vi "OAT Compensate Even Angle Signal (Even Angle Ref, 1 Channel).vi"(0 "even-angle signal":cluster{"r0":dbl, "dr":dbl, "Y":dbl[]}={"r0"=0.0, "dr"=1.0, "Y"=[]} {"r0" format="%.2p"; "dr" format="%.2p"; "Y" format="%.2f"}, 2 "reset? (F)":bool, 5 "even-angle reference":cluster{"r0":dbl, "dr":dbl, "Y":dbl[]}={"r0"=0.0, "dr"=1.0, "Y"=[]} {"r0" format="%.2p"; "dr" format="%.2p"; "Y" format="%.2f"}, 7 "even-angle position info":T1, 9 "speed profile":T2 {"speed [RPM]" format="%.2f"; "time [s]" format="%.2f"}, 11 "error in (no error)":errorcluster) -> (4 "compensated even-angle signal":cluster{"r0":dbl, "dr":dbl, "Y":dbl[]}={"r0"=0.0, "dr"=1.0, "Y"=[]} {"r0" format="%.2p"; "dr" format="%.2p"; "Y" format="%.2f"}, 6 "actual even-angle reference":cluster{"r0":dbl, "dr":dbl, "Y":dbl[]}={"r0"=0.0, "dr"=1.0, "Y"=[]} {"r0" format="%.2p"; "dr" format="%.2p"; "Y" format="%.2f"}, 8 "even-angle position info out":T1, 15 "error out":errorcluster)   [LabVIEW 2017, in "SoundVib_RefDataProcess.lvlib"]
doc: "Compensates an even-angle signal. You can use the <B>compensated even-angle signal</B> output to display unfiltered orbit and timebase plots with the runout pattern removed. Wire data to the <B>even-angle signal</B> input to determine the polymorphic instance to use or manually select the instance."
uses:
  <vilib>/addons/Sound and Vibration/Order Analysis/Referece Data Processing/SoundVib_RefDataProcess.lvlib
  <vilib>/addons/Sound and Vibration/Order Analysis/Misc/OAT Position Info.ctl
  <vilib>/addons/Sound and Vibration/Order Analysis/Tach Process/SubVIs/speed profile.ctl
  <vilib>/addons/Sound and Vibration/Order Analysis/Resample Order Tracking/SoundVib_Resampling.lvlib
  <vilib>/addons/Sound and Vibration/Order Analysis/Tach Process/SoundVib_TachProcess.lvlib
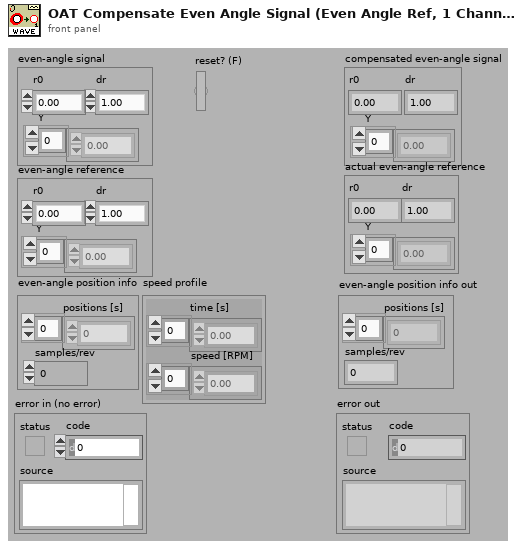
[diagram p1: front panel]
types:
  T1 = typedef "OAT Position Info.ctl" = cluster{"positions [s]":dbl[], "samples/rev":dbl}
  T2 = typedef "SoundVib_TachProcess.lvlib/speed profile.ctl" = cluster{"time [s]":dbl[], "speed [RPM]":dbl[]}
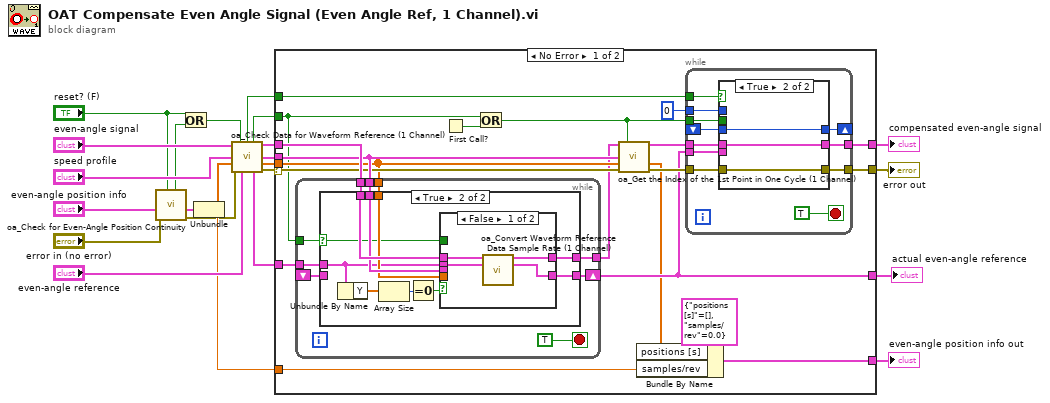
[diagram p0: block diagram]
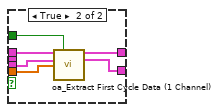
[diagram p3: hidden frame]
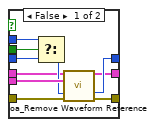
[diagram p4: hidden frame]
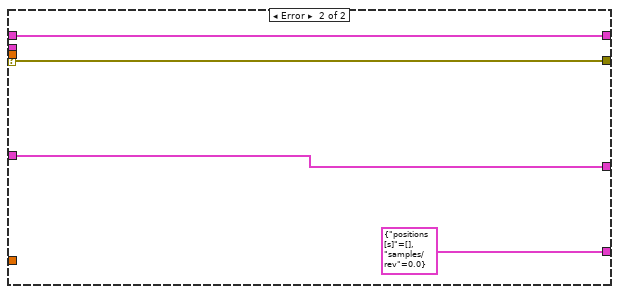
[diagram p5: hidden frame]
diagram:
  n1 = call <vilib>:"oa_Check for Even-Angle Position Continuity.vi"("reset in"="reset? (F)", "error in (no error)"="error in (no error)", "even-angle position info"="even-angle position info") -> ("error out"=w6:errorcluster, "even-angle position info dup"=w5:T1, "position not continuous"=w2:bool)  [unwired: 6 in]
  n2 = Or(x="reset? (F)", y=w2) -> (x .or. y?=w1:bool)
  n3 = Unbundle(w5) -> ("positions [s]"=w14:dbl[], "samples/rev"=w9:dbl)
  n4 = call <vilib>:"oa_Check Data for Waveform Reference (1 Channel).vi"("resampled signal"="even-angle signal", "reset? (True)"=w1, "speed profile"="speed profile", "interpolated pulse positions"=w14, "error in (no error)"=w6, "even angle reference in"="even-angle reference") -> ("empty signal?"=w10:bool, "reset"=w13:bool, "resampled signal out"=w20:cluster{"r0":dbl, "dr":dbl, "Y":dbl[]}, "speed profile out"=w19:T2, "interpolated pulse positions out"=w18:dbl[], "even angle reference out"=w11:cluster{"r0":dbl, "dr":dbl, "Y":dbl[]}, "error out"=w21:errorcluster)  [unwired: 2 in, 1 out]
  n5 = case shown="No Error" w21 {
    selector: w21 -> [w41 w102]
    tunnel: w20 -> [w43 w101]
    tunnel: w19 -> [w42 _]
    tunnel: w18 -> [w35 _]
    tunnel: [w37 w101] -> w17
    tunnel: [w34 w100] -> w16
    tunnel: [w38 w102] -> w15
    tunnel: w13 -> [w32 _]
    tunnel: w11 -> [w30 w100]
    tunnel: w10 -> [w29 _]
    tunnel: w9 -> [w27 _]
    tunnel: [w25 T1 {"positions [s]"=[], "samples/rev"=0.0} ("even angle position info")] -> w8
    frame No Error {
      n6 = while {
        tunnel: w43 -> [w52]
        tunnel: w42 -> [w51]
        tunnel: w32 -> [w46]
        tunnel: [w50] -> w24
        tunnel: w35 -> [w49]
        shift-right: [w47] -> w34
        shift-left: _ -> [w45]
        tunnel: w30 -> [w44]
        stop <- TRUE stop-if-true
        n7 = case shown="True" w46 {
          selector: w46 -> [_ w56]
          tunnel: w52 -> [w53 w64]
          tunnel: w51 -> [_ w63]
          tunnel: [w53 w59] -> w50
          tunnel: w49 -> [_ w58]
          tunnel: [w54 w57] -> w47
          tunnel: w45 -> [w54 _]
          tunnel: w44 -> [_ w55]
          frame False {
          }
          frame True {
            n8 = Unbundle By Name(w55) -> ("Y"=w62:dbl[])
            n9 = Array Size(array=w62) -> (size(s)=w61:i32)
            n10 = Equal To 0?(x=w61) -> (x = 0?=w60:bool)
            n11 = case shown="False" w60 {
              tunnel: w55 -> [w67 _]
              tunnel: [w66 w69] -> w57
              tunnel: w64 -> [w68 w74]
              tunnel: w56 -> [_ w73]
              tunnel: w63 -> [_ w72]
              tunnel: [w65 w70] -> w59
              tunnel: w58 -> [_ w71]
              frame False {
                n12 = call <vilib>:"oa_Convert Waveform Reference Data Sample Rate (1 Channel).vi"("resampled signal"=w68, "baseline in"=w67) -> ("resampled signal dup"=w65:cluster{"r0":dbl, "dr":dbl, "Y":dbl[]}, "baseline in out"=w66:cluster{"r0":dbl, "dr":dbl, "Y":dbl[]})  [unwired: 11 in, 1 out]
              }
              frame True {
                n13 = call <vilib>:"oa_Extract First Cycle Data (1 Channel).vi"("resampled signal"=w74, "reset? (True)"=w73, "speed profile"=w72, "interpolated pulse positions"=w71) -> ("resampled signal out"=w70:cluster{"r0":dbl, "dr":dbl, "Y":dbl[]}, "waveform reference data"=w69:cluster{"r0":dbl, "dr":dbl, "Y":dbl[]})  [unwired: 9 in, 1 out]
              }
            }
          }
        }
      }
      n14 = First Call?() -> (First Call?: T/F=w31:bool)
      n15 = Or(x=w32, y=w31) -> (x .or. y?=w33:bool)
      n16 = call <vilib>:"oa_Get the Index of the 1st Point in One Cycle (1 Channel).vi"("resampled signal"=w24, "reset? (True)"=w33, "speed profile"=w42, "interpolated pulse positions"=w35, "error in (no error)"=w41) -> ("resampled signal out"=w39:cluster{"r0":dbl, "dr":dbl, "Y":dbl[]}, "interpolated pulse positions out"=w26:dbl[], "error out"=w40:errorcluster)  [unwired: 8 in]
      n17 = Bundle By Name(cluster=T1 {"positions [s]"=[], "samples/rev"=0.0} ("even angle position info"), "positions [s]"=w26, "samples/rev"=w27) -> (w25:T1)
      n18 = while {
        tunnel: w40 -> [w85]
        tunnel: [w84] -> w38
        tunnel: w34 -> [w82]
        shift-right: [w81] -> _
        shift-left: _ -> [w79]
        tunnel: w33 -> [w80]
        tunnel: 0 ("t") -> [w76]
        tunnel: w39 -> [w78]
        tunnel: [w77] -> w37
        tunnel: w29 -> [w75]
        stop <- TRUE stop-if-true
        n19 = case shown="True" w75 {
          tunnel: w85 -> [w95 w96]
          tunnel: [w94 w96] -> w84
          tunnel: w82 -> [w93 _]
          tunnel: [w92 w98] -> w81
          tunnel: w80 -> [w91 _]
          tunnel: w79 -> [w90 w98]
          tunnel: w78 -> [w88 w97]
          tunnel: [w87 w97] -> w77
          tunnel: w76 -> [w86 _]
          frame False {
            n20 = Select(t=w86, s=w91, f=w90) -> (s? t:f=w89:i32)
            n21 = call <vilib>:"oa_Remove Waveform Reference.vi"("resampled signal"=w88, "baseline in"=w93, "last index"=w89, "error out in"=w95) -> ("compensated signal"=w87:cluster{"r0":dbl, "dr":dbl, "Y":dbl[]}, "last index out"=w92:i32, "error out"=w94:errorcluster)  [unwired: 9 in]
          }
          frame True {
          }
        }
      }
    }
    frame Error {
    }
  }
  "compensated even-angle signal" <- w17
  "actual even-angle reference" <- w16
  "error out" <- w15
  "even-angle position info out" <- w8
